vi "JSON Minify - Tokenizer.vi"(8 "error in (no error)":errorcluster, 10 "JSON String":string) -> (0 "error out":errorcluster, 1 "offset past":i32[](array[numeric]), 2 "matches":string[](array[string]), 5 "Right Context":string[](array[string]), 7 "Left Context":string[](array[string]))   [LabVIEW 2020]
uses:
  <vilib>/regexp/Match Regular Expression.xnode
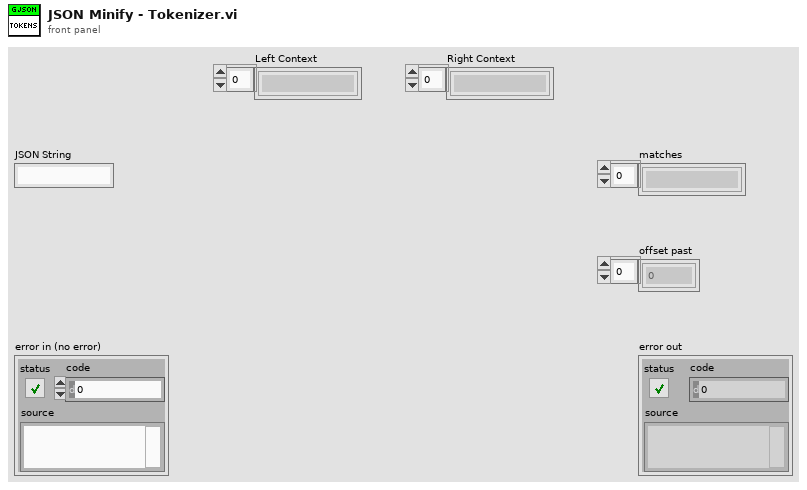
[diagram p1: front panel]
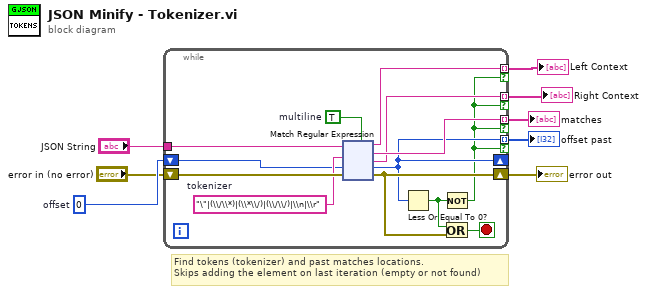
[diagram p0: block diagram]
diagram:
  w4 = 0  # offset
  # "Find tokens (tokenizer) and past matches locations.\nSkips adding the element on last iteration (empty or not found)"
  n1 = while {
    shift-right: [w17] -> w7
    shift-left: "error in (no error)" -> [w21]
    tunnel: "JSON String" -> [w20]
    tunnel: [w18] -> w5 mode=indexing if=w9
    tunnel: [w15] -> w8 mode=indexing if=w9
    shift-right: [w15] -> _
    shift-left: w4 -> [w14]
    tunnel: [w11] -> w2 mode=indexing if=w9
    tunnel: [w10] -> w1 mode=indexing if=w9
    stop <- w16 stop-if-true
    w12 = TRUE  # multiline
    w19 = "\"|(\\/\\*)|(\\*\\/)|(\\/\\/)|\\n|\\r"  # tokenizer
    n2 = xnode "Match Regular Expression"("input string"=w20, "regular expression"=w19, "offset (0)"=w14, "error in"=w21, "multiline? (F)"=w12) -> ("before match"=w11:string, "whole match"=w18:string, "after match"=w10:string, "offset past match"=w15:i32, "error out"=w17:errorcluster)  [unwired: 1 in]
    n3 = Less Or Equal To 0?(x=w15) -> (x <= 0?=w13:bool)
    n4 = Not(x=w13) -> (.not. x?=w9:bool)
    n5 = Or(x=w13, y=w17) -> (x .or. y?=w16:bool)
  }
  "offset past" <- w8
  "error out" <- w7
  "matches" <- w5
  "Left Context" <- w2
  "Right Context" <- w1
